vi "Read Dev.HardwareVersion.vi"(8 "error in (no error)":errorcluster, 11 "SLSC Remote in":refnum<class "SLSC Remote.lvclass">) -> (0 "error out":errorcluster, 2 "Dev.HardwareVersion":string, 3 "SLSC Remote out":refnum<class "SLSC Remote.lvclass">)   [LabVIEW 2016, in "SLSC Interfaces.lvlib" / "SLSC Remote.lvclass"]
uses:
  SLSC Remote.lvclass
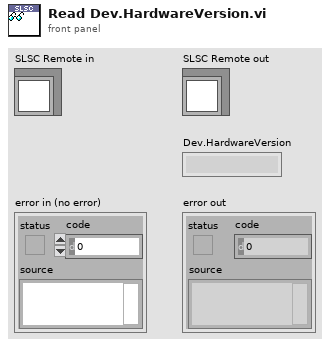
[diagram p1: front panel]
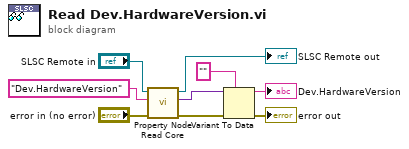
[diagram p0: block diagram]
diagram:
  n1 = call "Property Node Read Core.vi"("error in (no error)"="error in (no error)", "property"="Dev.HardwareVersion", "SLSC Remote in"="SLSC Remote in") -> ("error out"=w8:errorcluster, "value"=w9:variant, "SLSC Remote out"=→"SLSC Remote out":refnum<class "SLSC Remote.lvclass">)  [unwired: 6 in]
  n2 = Variant To Data(error in=w8, type="" ("Dev.HardwareVersion"), Variant=w9) -> (data=→"Dev.HardwareVersion":string, error out=→"error out":errorcluster)
